vi "pressure_regulator_test.vi"() -> ()   [LabVIEW 2019]
panel:
  out "Error":string
  out "Sensor output over time":dbl(graph)
  out "Sensor value (V)":dbl format="%.2f"
  in  "Sensor":string="AIN0"
  in  "stop":bool
  in  "FC value  (V)":dbl format="%.6f"
  in  "Flow controller":string="DAC0"
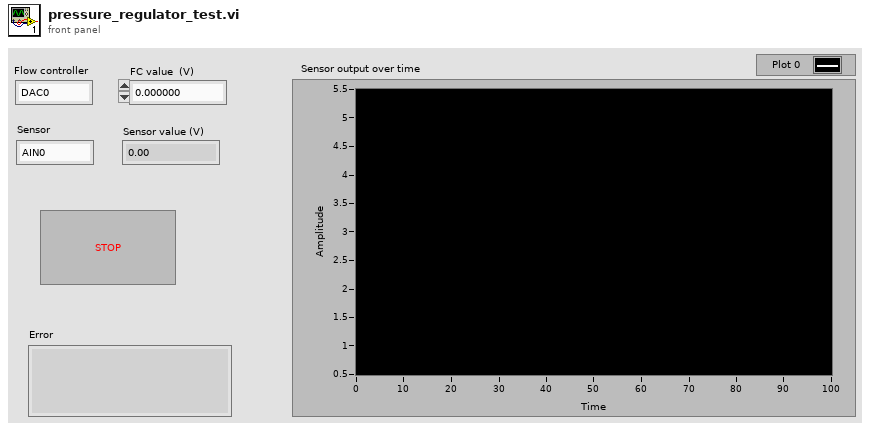
[diagram p1: front panel]
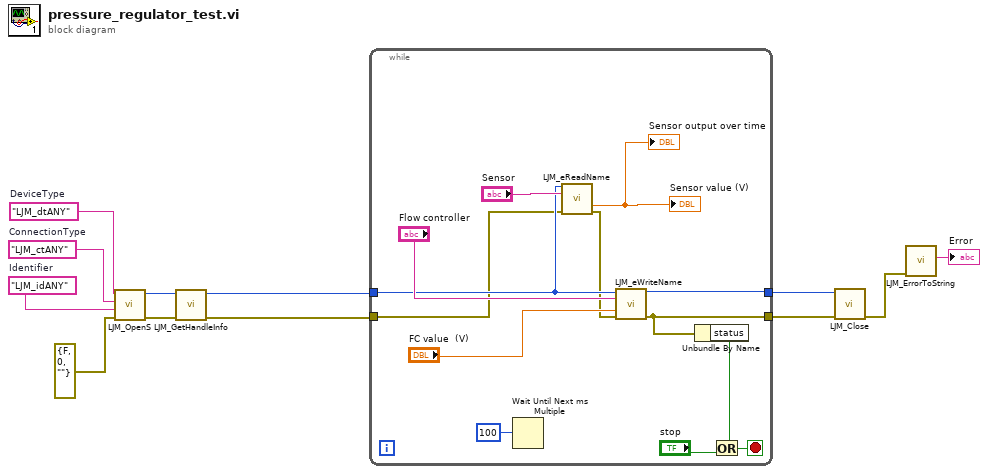
[diagram p0: block diagram]
diagram:
  w2 = "LJM_idANY"  # Identifier
  w3 = "LJM_ctANY"  # ConnectionType
  w4 = "LJM_dtANY"  # DeviceType
  n1 = call "LJM_OpenS.vi"("error in"=errorcluster {"status"=FALSE, "code"=0, "source"=""} ("error in (no error)"), "Identifier"=w2, "ConnectionType"=w3, "DeviceType"=w4) -> ("error out"=w11:errorcluster, "Handle"=w10:i32)  [unwired: 6 in]
  n2 = call "LJM_GetHandleInfo.vi"("error in"=w11, "Handle In"=w10) -> ("error out"=w5:errorcluster, "Handle Out"=w6:i32)  [unwired: 2 in, 6 out]
  n3 = while {
    tunnel: w5 -> [w15]
    tunnel: [w21] -> w8
    tunnel: w6 -> [w16]
    tunnel: [w22] -> w7
    stop <- w25 stop-if-true
    n4 = Wait Until Next ms Multiple(millisecond multiple=u32 100) -> ()  [unwired: 1 out]
    n5 = call "LJM_eReadName.vi"("Handle In"=w16, "Name"="Sensor", "error in"=w15) -> ("Value"=→"Sensor value (V)" →"Sensor output over time":dbl, "error out"=w14:errorcluster)  [unwired: 10 in, 1 out]
    n6 = call "LJM_eWriteName.vi"("Handle In"=w16, "Name"="Flow controller", "Value"="FC value  (V)", "error in"=w14) -> ("Handle Out"=w22:i32, "error out"=w21:errorcluster)  [unwired: 10 in]
    n7 = Unbundle By Name(w21) -> ("status"=w24:bool)
    n8 = Or(x=w24, y="stop") -> (x .or. y?=w25:bool)
  }
  n9 = call "LJM_Close.vi"("error in"=w8, "Handle"=w7) -> ("error out"=w9:errorcluster)  [unwired: 9 in]
  n10 = call "LJM_ErrorToString.vi"("error in"=w9) -> ("String"=→"Error":string)  [unwired: 10 in]
